vi "SaveOrLoadBeadlist.vi"(9 "beadlist filename":path, 10 "Load beadlist":bool, 11 "Bead locations (input)":cluster{"X":i32, "Y":i32}[](array[cluster])) -> (3 "Bead locations (output)":cluster{"X":i32, "Y":i32}[](array[cluster]))   [LabVIEW 2011]
uses:
  <vilib>/Utility/file.llb/Write To Spreadsheet File (I64).vi
  <vilib>/Utility/file.llb/Read From Spreadsheet File (DBL).vi
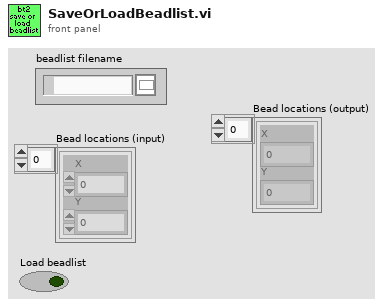
[diagram p1: front panel]
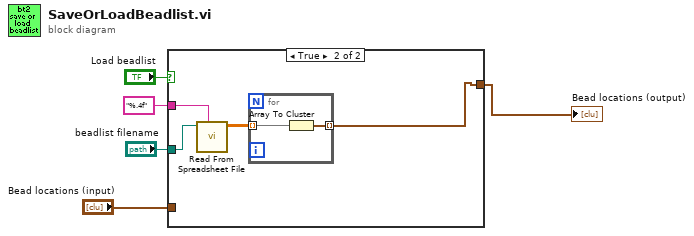
[diagram p0: block diagram]
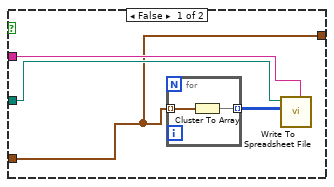
[diagram p2: hidden frame]
diagram:
  n1 = case shown="True" "Load beadlist" {
    tunnel: "beadlist filename" -> [w8 w15]
    tunnel: "%.4f" ("format (%.3f)") -> [w9 w13]
    tunnel: "Bead locations (input)" -> [w6 _]
    tunnel: [w6 w12] -> w1
    frame False {
      n2 = for {
        tunnel: w6 -> [w11] mode=indexing
        tunnel: [w10] -> w7 mode=indexing
        n3 = Cluster To Array(cluster=w11) -> (array=w10:i32[])
      }
      n4 = call-poly <vilib>:"Write To Spreadsheet File.vi"("format (%d)"=w9, "2D data"=w7, "file path (dialog if empty)"=w8) -> ()  [unwired: 3 in, 3 out]
    }
    frame True {
      n5 = call-poly <vilib>:"Read From Spreadsheet File.vi"("format (%.3f)"=w13, "file path (dialog if empty)"=w15) -> ("all rows"=w14:dbl[][])  [unwired: 5 in, 4 out]
      n6 = for {
        tunnel: w14 -> [w17] mode=indexing
        tunnel: [w16] -> w12 mode=indexing
        n7 = Array To Cluster(array=w17) -> (cluster=w16:cluster{"all rows[0]":dbl, "all rows[1]":dbl})
      }
    }
  }
  "Bead locations (output)" <- w1
